vi "createCommandList.vi"(8 "error in (no error)":errorcluster, 10 "Parameters":u32[](array[numeric]), 11 "Störaussendung in":refnum<class "Stoeraussendung.lvclass">) -> (0 "error out":errorcluster, 2 "Commandlist":string, 3 "Störaussendung out":refnum<class "Stoeraussendung.lvclass">)   [LabVIEW 2013, in "Stoeraussendung.lvclass"]
uses:
  Stoeraussendung.lvclass
  TestInterface/TestInterface.lvclass
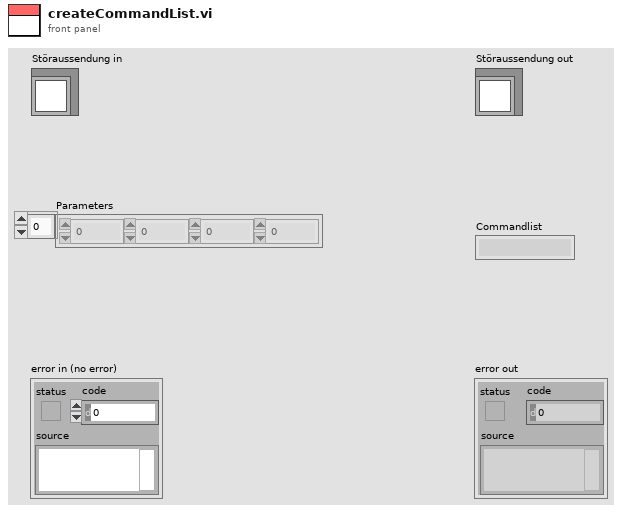
[diagram p1: front panel]
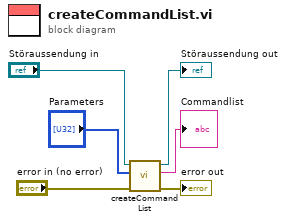
[diagram p0: block diagram]
diagram:
  n1 = call-parent "createCommandList.vi"("error in (no error)"="error in (no error)", "Parameters"="Parameters", "TestInterface in"="Störaussendung in") -> ("error out"=→"error out":errorcluster, "Commandlist"=→"Commandlist":string, "TestInterface out"=→"Störaussendung out":refnum<class "Stoeraussendung.lvclass">)  [unwired: 6 in]
